vi "Actualiza Mensaje.vi"(8 "error in (no error)":errorcluster, 10 "Mensaje Status":string, 11 "MENSAJES in":refnum<class "MENSAJES.lvclass">) -> (0 "error out":errorcluster, 3 "MENSAJES out":refnum<class "MENSAJES.lvclass">)   [LabVIEW 2019, in "MENSAJES.lvlib" / "MENSAJES.lvclass"]
uses:
  MENSAJES.lvclass
  MENSAJES.lvclass/MENSAJES.ctl
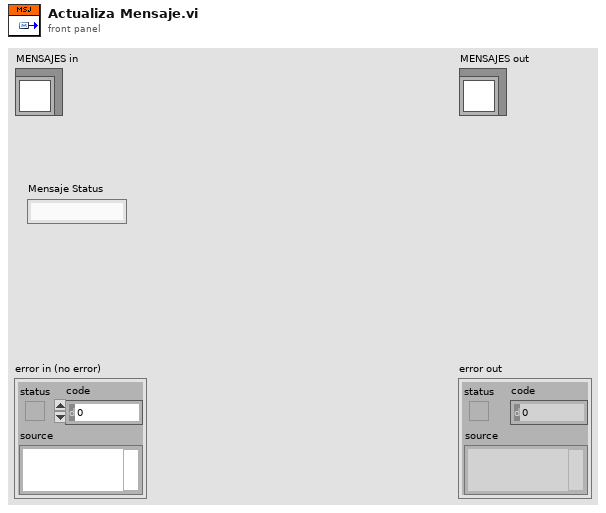
[diagram p1: front panel]
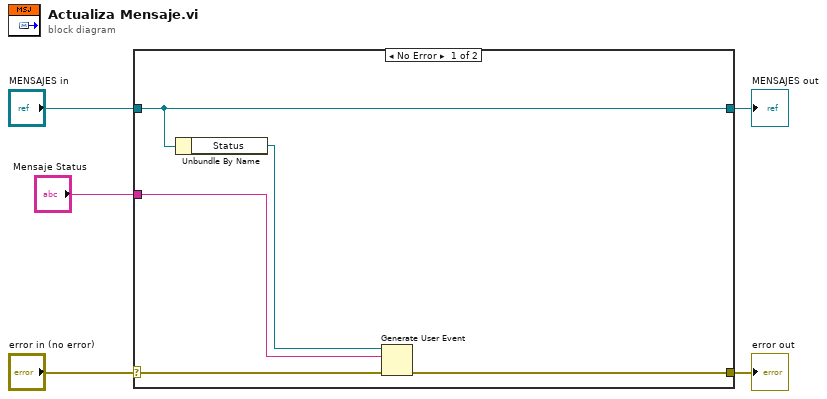
[diagram p0: block diagram]
diagram:
  n1 = case shown="No Error" "error in (no error)" {
    selector: "error in (no error)" -> [w9 w12]
    tunnel: [w8 w12] -> w4
    tunnel: [w10 w11] -> w2
    tunnel: "MENSAJES in" -> [w10 w11]
    tunnel: "Mensaje Status" -> [w6 _]
    frame No Error {
      n2 = Unbundle By Name(w10) -> ("Status"=w7:refnum<user-event>)
      n3 = Generate User Event(user event=w7, event data cluster=w6, error in=w9) -> (error out=w8:errorcluster)  [unwired: 1 in, 1 out]
    }
    frame Error {
    }
  }
  "error out" <- w4
  "MENSAJES out" <- w2
